vi "SDCP - Standard Message Frames Editor - Generate C code.vi"(2 "error in (no error)":errorcluster, 3 "Frame details":T2(array[cluster])) -> (0 "error out":errorcluster, 1 "Output":string)   [LabVIEW 2020]
uses:
  Typedefs/SDCP - Standard Message Frames Editor - Parameter cluster.ctl
panel:
  out "Array":string[](array[string])
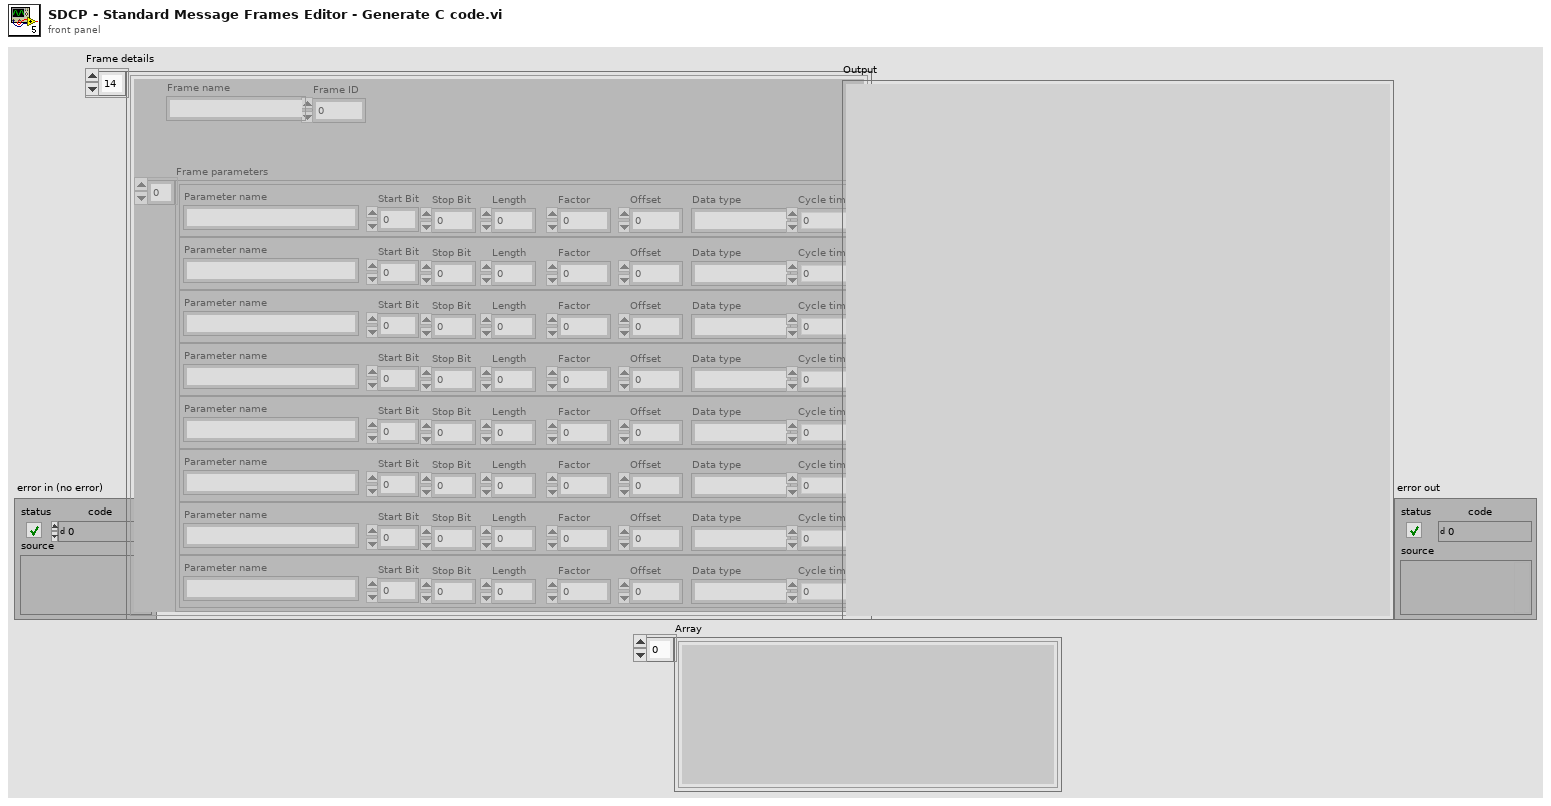
[diagram p1: front panel]
types:
  T1 = typedef "SDCP - Standard Message Frames Editor - Parameter cluster.ctl" = cluster{"Parameter name":string, "Start Bit":i32, "Stop Bit":i32, "Length":i32, "Factor":dbl, "Offset":dbl, "Data type":string, "Cycle time":dbl}
  T2 = cluster{"Frame name":string, "Frame ID":i32, "Frame parameters":T1[]}[]
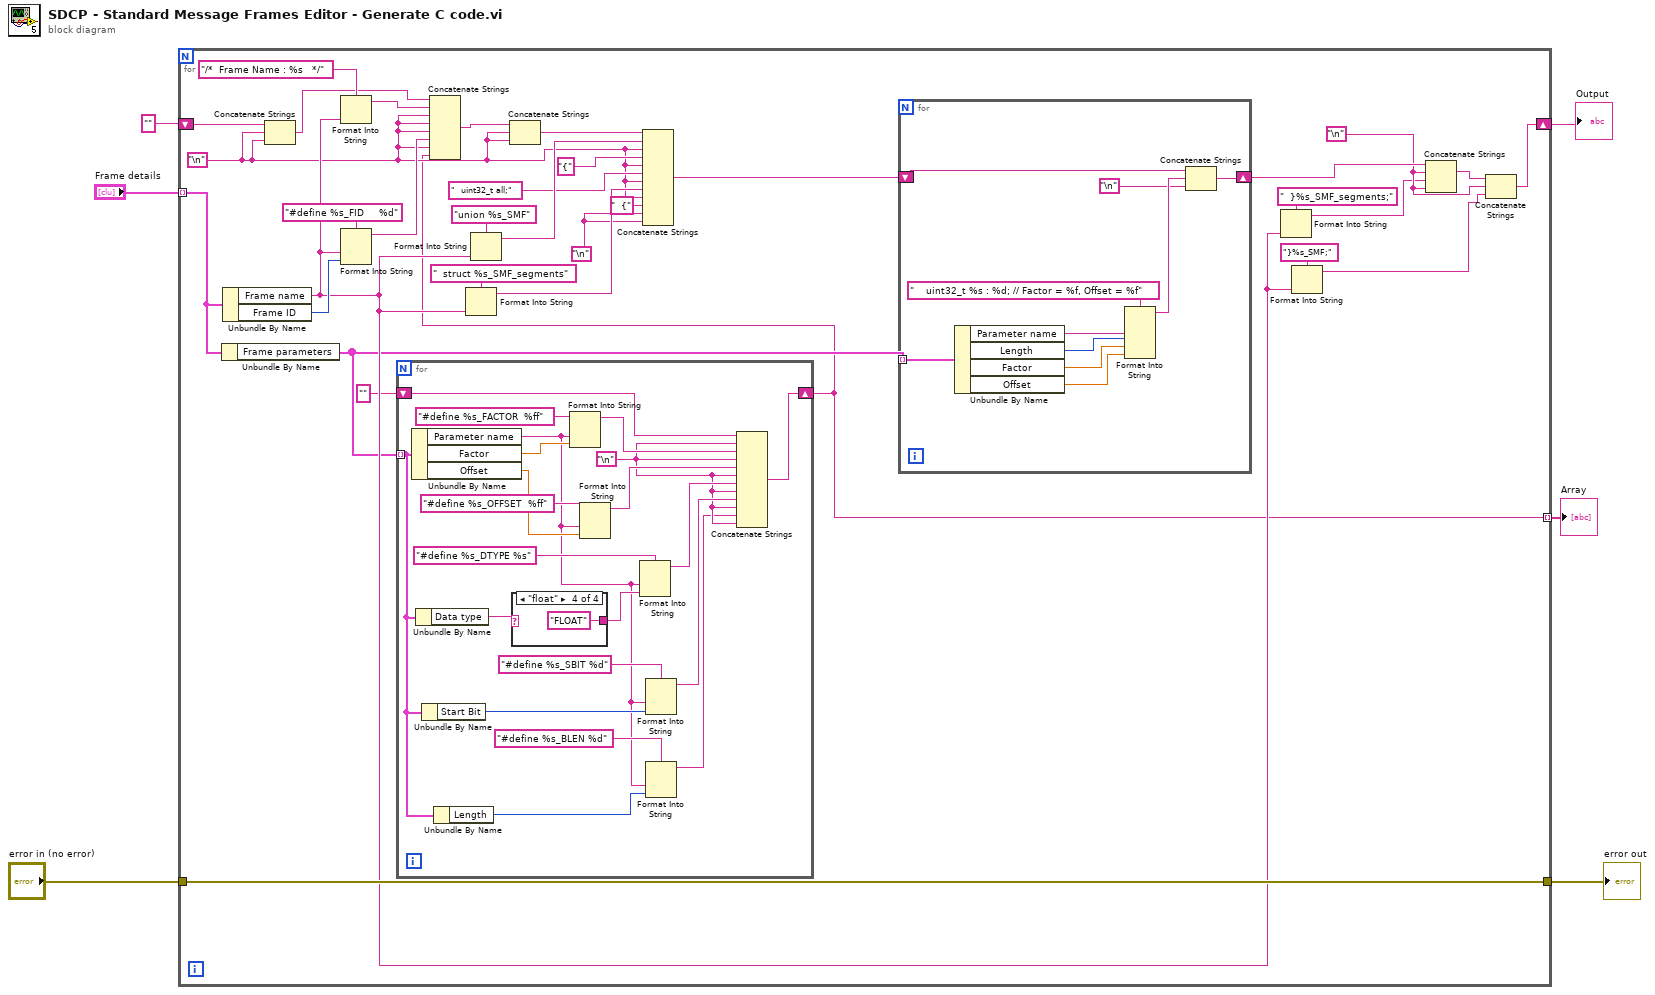
[diagram p0: block diagram]
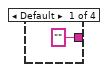
[diagram p2: hidden frame]
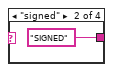
[diagram p3: hidden frame]
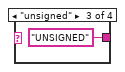
[diagram p4: hidden frame]
diagram:
  n1 = for {
    shift-right: [w19] -> w4
    shift-left: "" -> [w37]
    tunnel: "Frame details" -> [w24] mode=indexing
    tunnel: "error in (no error)" -> [w27]
    tunnel: [w27] -> w2
    tunnel: [w7] -> w1 mode=indexing
    w18 = "\n"
    w17 = "\n"
    w8 = "\n"
    n2 = Unbundle By Name(w24) -> ("Frame parameters"=w10:T1[])
    n3 = Unbundle By Name(w24) -> ("Frame name"=w12:string, "Frame ID"=w38:i32)
    n4 = Concatenate Strings(w37, w8, w8) -> (w11:string)
    n5 = Format Into String(format string="/*  Frame Name : %s   */", w12) -> (resulting string=w13:string)  [unwired: 2 in, 1 out]
    n6 = Format Into String(format string="#define %s_FID     %d", w12, w38) -> (resulting string=w36:string)  [unwired: 2 in, 1 out]
    n7 = for {
      tunnel: w10 -> [w42] mode=indexing
      shift-right: [w55] -> w7
      shift-left: "" -> [w54]
      w45 = "\n"
      n8 = Unbundle By Name(w42) -> ("Parameter name"=w43:string, "Factor"=w59:dbl, "Offset"=w57:dbl)
      n9 = Unbundle By Name(w42) -> ("Data type"=w51:string)
      n10 = Unbundle By Name(w42) -> ("Start Bit"=w47:i32)
      n11 = Unbundle By Name(w42) -> ("Length"=w41:i32)
      n12 = case shown="\"float\"" w51 {
        tunnel: ["" "SIGNED" "UNSIGNED" "FLOAT"] -> w50
        frame Default {
        }
        frame "signed" {
        }
        frame "unsigned" {
        }
        frame "float" {
        }
      }
      n13 = Format Into String(format string="#define %s_FACTOR  %ff", w43, w59) -> (resulting string=w58:string)  [unwired: 2 in, 1 out]
      n14 = Format Into String(format string="#define %s_OFFSET  %ff", w43, w57) -> (resulting string=w56:string)  [unwired: 2 in, 1 out]
      n15 = Format Into String(format string="#define %s_DTYPE %s", w43, w50) -> (resulting string=w49:string)  [unwired: 2 in, 1 out]
      n16 = Format Into String(format string="#define %s_SBIT %d", w43, w47) -> (resulting string=w46:string)  [unwired: 2 in, 1 out]
      n17 = Format Into String(format string="#define %s_BLEN %d", w43, w41) -> (resulting string=w40:string)  [unwired: 2 in, 1 out]
      n18 = Concatenate Strings(w54, w45, w58, w45, w56, w45, w49, w45, w46, w45, w40, w45) -> (w55:string)
    }
    n19 = Concatenate Strings(w11, w13, w8, w8, w8, w36, w8, w7) -> (w35:string)
    n20 = Format Into String(format string="  struct %s_SMF_segments", w12) -> (resulting string=w29:string)  [unwired: 2 in, 1 out]
    n21 = Format Into String(format string="union %s_SMF", w12) -> (resulting string=w32:string)  [unwired: 2 in, 1 out]
    n22 = Concatenate Strings(w35, w8, w8) -> (w34:string)
    n23 = Concatenate Strings(w34, w32, w8, "{" ("string"), w8, "  uint32_t all;" ("string"), w8, w29, w8, "  {" ("string"), w18, w18) -> (w25:string)
    n24 = for {
      shift-right: [w65] -> w23
      shift-left: w25 -> [w68]
      tunnel: w10 -> [w73] mode=indexing
      n25 = Unbundle By Name(w73) -> ("Parameter name"=w72:string, "Length"=w71:i32, "Factor"=w70:dbl, "Offset"=w69:dbl)
      n26 = Format Into String(format string="    uint32_t %s : %d; // Factor = %f, Offset = %f", w72, w71, w70, w69) -> (resulting string=w67:string)  [unwired: 2 in, 1 out]
      n27 = Concatenate Strings(w68, w67, "\n") -> (w65:string)
    }
    n28 = Format Into String(format string="  }%s_SMF_segments;", w12) -> (resulting string=w16:string)  [unwired: 2 in, 1 out]
    n29 = Format Into String(format string="}%s_SMF;", w12) -> (resulting string=w15:string)  [unwired: 2 in, 1 out]
    n30 = Concatenate Strings(w23, w17, w16, w17) -> (w21:string)
    n31 = Concatenate Strings(w21, w17, w15) -> (w19:string)
  }
  "error out" <- w2
  "Output" <- w4
  "Array" <- w1
